vi "Lab Panel V5.11.vi"() -> ()   [LabVIEW 2013] (continued)
                            n1494 = local write "DISP LAB05-2"(w2804) -> ()
                          }
                        }
                      }
                      frame False {
                      }
                    }
                  }
                }
              }
            }
          }
          frame #6 {
            # "end test & close test files"
            n1495 = local read "MAIL SETTINGS"() -> (w2810:T7)
            n1496 = Unbundle(w2810) -> ("OUT SERVER ADDRESS"=w2809:string, "FROM ACCOUNT"=w2808:string)  [unwired: 5 out]
            n1497 = stacked-sequence {
              tunnel: w2820 -> [_ _ _ _ _ _ _ _ _ _]
              tunnel: w2821 -> [_ _ _ _ _ _ _ _ _ _]
              tunnel: w2819 -> [_ _ _ _ _ _ _ _ _ _]
              tunnel: w2818 -> [_ _ _ _ _ _ _ _ _ _]
              tunnel: w2817 -> [_ _ _ _ _ _ _ _ _ _]
              tunnel: w2816 -> [_ _ _ _ _ _ _ _ _ _]
              tunnel: w2815 -> [_ _ _ _ _ _ _ _ _ _]
              tunnel: w2814 -> [_ _ _ _ _ _ _ _ _ _]
              tunnel: w2813 -> [_ _ _ _ _ _ _ _ _ _]
              tunnel: w2812 -> [_ _ _ _ _ _ _ _ _ _]
              tunnel: w2809 -> [w2825 w2877 w2925 w2972 w3019 w3066 w3113 w3160 w3207 w3254]
              tunnel: w2808 -> [w2824 w2876 w2924 w2971 w3018 w3065 w3112 w3159 w3206 w3253]
              tunnel: "Mail Test File To:" -> [w2823 w2875 w2923 w2970 w3017 w3064 w3111 w3158 w3205 w3252]
              tunnel: "Mail Test Fail" -> [w2822 w2874 w2922 w2969 w3016 w3063 w3110 w3157 w3204 w3251]
              frame #0 {
                # "LAB01-1"
                n1498 = local read "DISP LAB01-1"() -> (w2829:T4)
                n1499 = local read "run lab01-1"() -> (w2826:bool)
                n1500 = local read "TDMS LAB01-1"() -> (w2827:refnum<k34>)
                n1501 = Unbundle(w2829) -> ("CYCLE"=w2830:dbl, "STATUS"=w2828:string)  [unwired: 1 out]
                n1502 = case shown="True" w2826 {
                  tunnel: w2830 -> [_ w2836]
                  tunnel: w2829 -> [_ w2838]
                  tunnel: w2828 -> [_ w2835]
                  tunnel: w2827 -> [_ w2837]
                  tunnel: w2825 -> [_ w2834]
                  tunnel: w2824 -> [_ w2833]
                  tunnel: w2823 -> [_ w2832]
                  tunnel: w2822 -> [_ w2831]
                  frame False {
                  }
                  frame True {
                    n1503 = Not Equal?(x=w2835, y="RUN") -> (x != y?=w2839:bool)
                    n1504 = Greater?(x=w2836, y=2.0) -> (0:w2841:bool)
                    n1505 = And(x=w2841, y=w2839) -> (x .and. y?=w2840:bool)
                    n1506 = case shown="True" w2840 {
                      tunnel: w2838 -> [_ w2851]
                      tunnel: w2837 -> [_ w2850]
                      tunnel: w2836 -> [_ w2849]
                      tunnel: w2835 -> [_ w2848]
                      tunnel: w2834 -> [_ w2847]
                      tunnel: w2833 -> [_ w2846]
                      tunnel: w2832 -> [_ w2845]
                      tunnel: w2831 -> [_ w2844]
                      frame False {
                      }
                      frame True {
                        n1507 = stacked-sequence {
                          tunnel: w2851 -> [w2855 _ _]
                          tunnel: w2850 -> [_ w2857 _]
                          tunnel: w2849 -> [_ _ _]
                          tunnel: w2848 -> [_ _ w2863]
                          tunnel: w2847 -> [_ _ w2862]
                          tunnel: w2846 -> [_ _ w2861]
                          tunnel: w2845 -> [_ _ w2860]
                          tunnel: w2844 -> [_ _ w2859]
                          frame #0 {
                            w2852 = FALSE
                            n1508 = local write "mail control"("END") -> ()
                            n1509 = Bundle(cluster=w2855) -> (w2854:T4)  [unwired: 3 in]
                            n1510 = local write "DISP LAB01-1"(w2854) -> ()
                            n1511 = local write "O/I  LAB01-1"(w2852) -> ()
                            n1512 = local write "run lab01-1"(w2852) -> ()
                            n1513 = local write "RUN LAB01-1"(w2852) -> ()
                          }
                          frame #1 {
                            n1514 = TDMS Close(11:w2857) -> (0:w2856:errorcluster)  [unwired: 1 in, 1 out]
                            n1515 = local write "data file error"(w2856) -> ()
                          }
                          frame #2 {
                            n1516 = stacked-sequence {
                              tunnel: "LAB01-1" -> [w2865 w2867 _]
                              tunnel: w2863 -> [_ w2873 _]
                              tunnel: w2862 -> [_ w2872 _]
                              tunnel: w2861 -> [_ w2871 _]
                              tunnel: w2860 -> [_ w2870 _]
                              tunnel: w2859 -> [_ w2869 _]
                              frame #0 {
                                n1517 = call "sub vi - defrag tdms v1.vi"("panel id"=w2865) -> ("error out"=w2864:errorcluster)  [unwired: 10 in]
                                n1518 = local write "data file error"(w2864) -> ()
                              }
                              frame #1 {
                                n1519 = Bundle("STATUS"=w2873, "OUT SERVER ADDRESS"=w2872, "FROM ACCOUNT"=w2871, "Mail Test File To:"=w2870, "Mail Test Fail"=w2869) -> (w2866:T25)  [unwired: 1 in]
                                n1520 = call "Save data file (pass-fail) v5.vi"("Input Cluster"=w2866, "panel id"=w2867) -> ("network file save error"=w2868:errorcluster)  [unwired: 8 in, 1 out]
                                n1521 = local write "data file error"(w2868) -> ()
                              }
                              frame #2 {
                              }
                            }
                          }
                        }
                      }
                    }
                  }
                }
              }
              frame #1 {
                # "LAB01-2"
                n1522 = local read "run lab01-2"() -> (w2878:bool)
                n1523 = case shown="True" w2878 {
                  tunnel: w2877 -> [_ w2882]
                  tunnel: w2876 -> [_ w2881]
                  tunnel: w2875 -> [_ w2880]
                  tunnel: w2874 -> [_ w2879]
                  frame False {
                  }
                  frame True {
                    n1524 = local read "DISP LAB01-2"() -> (w2890:T4)
                    n1525 = local read "TDMS LAB01-2"() -> (w2889:refnum<k34>)
                    n1526 = Unbundle(w2890) -> ("CYCLE"=w2884:dbl, "STATUS"=w2883:string)  [unwired: 1 out]
                    n1527 = Not Equal?(x=w2883, y="RUN") -> (x != y?=w2886:bool)
                    n1528 = Greater?(x=w2884, y=2.0) -> (0:w2887:bool)
                    n1529 = And(x=w2887, y=w2886) -> (x .and. y?=w2885:bool)
                    n1530 = case shown="True" w2885 {
                      tunnel: w2890 -> [_ w2899]
                      tunnel: w2889 -> [_ w2898]
                      tunnel: w2884 -> [_ w2897]
                      tunnel: w2883 -> [_ w2896]
                      tunnel: w2882 -> [_ w2895]
                      tunnel: w2881 -> [_ w2894]
                      tunnel: w2880 -> [_ w2893]
                      tunnel: w2879 -> [_ w2892]
                      frame False {
                      }
                      frame True {
                        n1531 = stacked-sequence {
                          tunnel: w2899 -> [w2902 _ _]
                          tunnel: w2898 -> [_ w2904 _]
                          tunnel: w2897 -> [_ _ _]
                          tunnel: w2896 -> [_ _ w2910]
                          tunnel: w2895 -> [_ _ w2909]
                          tunnel: w2894 -> [_ _ w2908]
                          tunnel: w2893 -> [_ _ w2907]
                          tunnel: w2892 -> [_ _ w2906]
                          frame #0 {
                            w2900 = FALSE
                            n1532 = local write "mail control"("END") -> ()
                            n1533 = Bundle(cluster=w2902) -> (w2903:T4)  [unwired: 3 in]
                            n1534 = local write "RUN LAB01-2"(w2900) -> ()
                            n1535 = local write "run lab01-2"(w2900) -> ()
                            n1536 = local write "O/I  LAB01-2"(w2900) -> ()
                            n1537 = local write "DISP LAB01-2"(w2903) -> ()
                          }
                          frame #1 {
                            n1538 = TDMS Close(11:w2904) -> (0:w2905:errorcluster)  [unwired: 1 in, 1 out]
                            n1539 = local write "data file error"(w2905) -> ()
                          }
                          frame #2 {
                            n1540 = stacked-sequence {
                              tunnel: "LAB01-2" -> [w2913 w2914]
                              tunnel: w2910 -> [_ w2919]
                              tunnel: w2909 -> [_ w2918]
                              tunnel: w2908 -> [_ w2917]
                              tunnel: w2907 -> [_ w2916]
                              tunnel: w2906 -> [_ w2915]
                              frame #0 {
                                n1541 = call "sub vi - defrag tdms v1.vi"("panel id"=w2913) -> ("error out"=w2912:errorcluster)  [unwired: 10 in]
                                n1542 = local write "data file error"(w2912) -> ()
                              }
                              frame #1 {
                                n1543 = Bundle("STATUS"=w2919, "OUT SERVER ADDRESS"=w2918, "FROM ACCOUNT"=w2917, "Mail Test File To:"=w2916, "Mail Test Fail"=w2915) -> (w2921:T25)  [unwired: 1 in]
                                n1544 = call "Save data file (pass-fail) v5.vi"("Input Cluster"=w2921, "panel id"=w2914) -> ("network file save error"=w2920:errorcluster)  [unwired: 8 in, 1 out]
                                n1545 = local write "data file error"(w2920) -> ()
                              }
                            }
                          }
                        }
                      }
                    }
                  }
                }
              }
              frame #2 {
                # "LAB02-1"
                n1546 = local read "run lab02-1"() -> (w2926:bool)
                n1547 = case shown="True" w2926 {
                  tunnel: w2925 -> [_ w2930]
                  tunnel: w2924 -> [_ w2929]
                  tunnel: w2923 -> [_ w2928]
                  tunnel: w2922 -> [_ w2927]
                  frame False {
                  }
                  frame True {
                    n1548 = local read "DISP LAB02-1"() -> (w2938:T4)
                    n1549 = Unbundle(w2938) -> ("CYCLE"=w2934:dbl, "STATUS"=w2931:string)  [unwired: 1 out]
                    n1550 = local read "TDMS LAB02-1"() -> (w2937:refnum<k34>)
                    n1551 = Not Equal?(x=w2931, y="RUN") -> (x != y?=w2933:bool)
                    n1552 = Greater?(x=w2934, y=2.0) -> (0:w2935:bool)
                    n1553 = And(x=w2935, y=w2933) -> (x .and. y?=w2932:bool)
                    n1554 = case shown="True" w2932 {
                      tunnel: w2938 -> [_ w2946]
                      tunnel: w2937 -> [_ w2945]
                      tunnel: w2931 -> [_ w2944]
                      tunnel: w2930 -> [_ w2943]
                      tunnel: w2929 -> [_ w2942]
                      tunnel: w2928 -> [_ w2941]
                      tunnel: w2927 -> [_ w2940]
                      frame False {
                      }
                      frame True {
                        n1555 = stacked-sequence {
                          tunnel: w2946 -> [w2949 _ _]
                          tunnel: w2945 -> [_ w2951 _]
                          tunnel: w2944 -> [_ _ w2957]
                          tunnel: w2943 -> [_ _ w2956]
                          tunnel: w2942 -> [_ _ w2955]
                          tunnel: w2941 -> [_ _ w2954]
                          tunnel: w2940 -> [_ _ w2953]
                          frame #0 {
                            w2947 = FALSE
                            n1556 = local write "mail control"("END") -> ()
                            n1557 = Bundle(cluster=w2949) -> (w2950:T4)  [unwired: 3 in]
                            n1558 = local write "O/I  LAB02-1"(w2947) -> ()
                            n1559 = local write "RUN LAB02-1"(w2947) -> ()
                            n1560 = local write "run lab02-1"(w2947) -> ()
                            n1561 = local write "DISP LAB02-1"(w2950) -> ()
                          }
                          frame #1 {
                            n1562 = TDMS Close(11:w2951) -> (0:w2952:errorcluster)  [unwired: 1 in, 1 out]
                            n1563 = local write "data file error"(w2952) -> ()
                          }
                          frame #2 {
                            n1564 = stacked-sequence {
                              tunnel: "LAB02-1" -> [w2960 w2967]
                              tunnel: w2957 -> [_ w2965]
                              tunnel: w2956 -> [_ w2964]
                              tunnel: w2955 -> [_ w2963]
                              tunnel: w2954 -> [_ w2962]
                              tunnel: w2953 -> [_ w2961]
                              frame #0 {
                                n1565 = call "sub vi - defrag tdms v1.vi"("panel id"=w2960) -> ("error out"=w2959:errorcluster)  [unwired: 10 in]
                                n1566 = local write "data file error"(w2959) -> ()
                              }
                              frame #1 {
                                n1567 = Bundle("STATUS"=w2965, "OUT SERVER ADDRESS"=w2964, "FROM ACCOUNT"=w2963, "Mail Test File To:"=w2962, "Mail Test Fail"=w2961) -> (w2966:T25)  [unwired: 1 in]
                                n1568 = call "Save data file (pass-fail) v5.vi"("Input Cluster"=w2966, "panel id"=w2967) -> ("network file save error"=w2968:errorcluster)  [unwired: 8 in, 1 out]
                                n1569 = local write "data file error"(w2968) -> ()
                              }
                            }
                          }
                        }
                      }
                    }
                  }
                }
              }
              frame #3 {
                # "LAB02-2"
                n1570 = local read "run lab02-2"() -> (w2973:bool)
                n1571 = case shown="True" w2973 {
                  tunnel: w2972 -> [_ w2977]
                  tunnel: w2971 -> [_ w2976]
                  tunnel: w2970 -> [_ w2975]
                  tunnel: w2969 -> [_ w2974]
                  frame False {
                  }
                  frame True {
                    n1572 = local read "DISP LAB02-2"() -> (w2985:T4)
                    n1573 = local read "TDMS LAB02-2"() -> (w2984:refnum<k34>)
                    n1574 = Unbundle(w2985) -> ("CYCLE"=w2981:dbl, "STATUS"=w2978:string)  [unwired: 1 out]
                    n1575 = Not Equal?(x=w2978, y="RUN") -> (x != y?=w2980:bool)
                    n1576 = Greater?(x=w2981, y=2.0) -> (0:w2982:bool)
                    n1577 = And(x=w2982, y=w2980) -> (x .and. y?=w2979:bool)
                    n1578 = case shown="True" w2979 {
                      tunnel: w2985 -> [_ w2993]
                      tunnel: w2984 -> [_ w2992]
                      tunnel: w2978 -> [_ w2991]
                      tunnel: w2977 -> [_ w2990]
                      tunnel: w2976 -> [_ w2989]
                      tunnel: w2975 -> [_ w2988]
                      tunnel: w2974 -> [_ w2987]
                      frame False {
                      }
                      frame True {
                        n1579 = stacked-sequence {
                          tunnel: w2993 -> [w2996 _ _]
                          tunnel: w2992 -> [_ w2998 _]
                          tunnel: w2991 -> [_ _ w3004]
                          tunnel: w2990 -> [_ _ w3003]
                          tunnel: w2989 -> [_ _ w3002]
                          tunnel: w2988 -> [_ _ w3001]
                          tunnel: w2987 -> [_ _ w3000]
                          frame #0 {
                            w2994 = FALSE
                            n1580 = local write "mail control"("END") -> ()
                            n1581 = Bundle(cluster=w2996) -> (w2997:T4)  [unwired: 3 in]
                            n1582 = local write "O/I  LAB02-2"(w2994) -> ()
                            n1583 = local write "run lab02-2"(w2994) -> ()
                            n1584 = local write "RUN LAB02-2"(w2994) -> ()
                            n1585 = local write "DISP LAB02-2"(w2997) -> ()
                          }
                          frame #1 {
                            n1586 = TDMS Close(11:w2998) -> (0:w2999:errorcluster)  [unwired: 1 in, 1 out]
                            n1587 = local write "data file error"(w2999) -> ()
                          }
                          frame #2 {
                            n1588 = stacked-sequence {
                              tunnel: "LAB02-2" -> [w3007 w3013]
                              tunnel: w3004 -> [_ w3012]
                              tunnel: w3003 -> [_ w3011]
                              tunnel: w3002 -> [_ w3010]
                              tunnel: w3001 -> [_ w3009]
                              tunnel: w3000 -> [_ w3008]
                              frame #0 {
                                n1589 = call "sub vi - defrag tdms v1.vi"("panel id"=w3007) -> ("error out"=w3006:errorcluster)  [unwired: 10 in]
                                n1590 = local write "data file error"(w3006) -> ()
                              }
                              frame #1 {
                                n1591 = Bundle("STATUS"=w3012, "OUT SERVER ADDRESS"=w3011, "FROM ACCOUNT"=w3010, "Mail Test File To:"=w3009, "Mail Test Fail"=w3008) -> (w3015:T25)  [unwired: 1 in]
                                n1592 = call "Save data file (pass-fail) v5.vi"("Input Cluster"=w3015, "panel id"=w3013) -> ("network file save error"=w3014:errorcluster)  [unwired: 8 in, 1 out]
                                n1593 = local write "data file error"(w3014) -> ()
                              }
                            }
                          }
                        }
                      }
                    }
                  }
                }
              }
              frame #4 {
                # "LAB03-1"
                n1594 = local read "run lab03-1"() -> (w3020:bool)
                n1595 = case shown="True" w3020 {
                  tunnel: w3019 -> [_ w3024]
                  tunnel: w3018 -> [_ w3023]
                  tunnel: w3017 -> [_ w3022]
                  tunnel: w3016 -> [_ w3021]
                  frame False {
                  }
                  frame True {
                    n1596 = local read "DISP LAB03-1"() -> (w3032:T4)
                    n1597 = local read "TDMS LAB03-1"() -> (w3031:refnum<k34>)
                    n1598 = Unbundle(w3032) -> ("CYCLE"=w3028:dbl, "STATUS"=w3025:string)  [unwired: 1 out]
                    n1599 = Not Equal?(x=w3025, y="RUN") -> (x != y?=w3027:bool)
                    n1600 = Greater?(x=w3028, y=2.0) -> (0:w3029:bool)
                    n1601 = And(x=w3029, y=w3027) -> (x .and. y?=w3026:bool)
                    n1602 = case shown="True" w3026 {
                      tunnel: w3032 -> [_ w3040]
                      tunnel: w3031 -> [_ w3039]
                      tunnel: w3025 -> [_ w3038]
                      tunnel: w3024 -> [_ w3037]
                      tunnel: w3023 -> [_ w3036]
                      tunnel: w3022 -> [_ w3035]
                      tunnel: w3021 -> [_ w3034]
                      frame False {
                      }
                      frame True {
                        n1603 = stacked-sequence {
                          tunnel: w3040 -> [w3043 _ _]
                          tunnel: w3039 -> [_ w3045 _]
                          tunnel: w3038 -> [_ _ w3051]
                          tunnel: w3037 -> [_ _ w3050]
                          tunnel: w3036 -> [_ _ w3049]
                          tunnel: w3035 -> [_ _ w3048]
                          tunnel: w3034 -> [_ _ w3047]
                          frame #0 {
                            w3041 = FALSE
                            n1604 = local write "mail control"("END") -> ()
                            n1605 = Bundle(cluster=w3043) -> (w3044:T4)  [unwired: 3 in]
                            n1606 = local write "O/I  LAB03-1"(w3041) -> ()
                            n1607 = local write "run lab03-1"(w3041) -> ()
                            n1608 = local write "RUN LAB03-1"(w3041) -> ()
                            n1609 = local write "DISP LAB03-1"(w3044) -> ()
                          }
                          frame #1 {
                            n1610 = TDMS Close(11:w3045) -> (0:w3046:errorcluster)  [unwired: 1 in, 1 out]
                            n1611 = local write "data file error"(w3046) -> ()
                          }
                          frame #2 {
                            n1612 = stacked-sequence {
                              tunnel: "LAB03-1" -> [w3054 w3060]
                              tunnel: w3051 -> [_ w3059]
                              tunnel: w3050 -> [_ w3058]
                              tunnel: w3049 -> [_ w3057]
                              tunnel: w3048 -> [_ w3056]
                              tunnel: w3047 -> [_ w3055]
                              frame #0 {
                                n1613 = call "sub vi - defrag tdms v1.vi"("panel id"=w3054) -> ("error out"=w3053:errorcluster)  [unwired: 10 in]
                                n1614 = local write "data file error"(w3053) -> ()
                              }
                              frame #1 {
                                n1615 = Bundle("STATUS"=w3059, "OUT SERVER ADDRESS"=w3058, "FROM ACCOUNT"=w3057, "Mail Test File To:"=w3056, "Mail Test Fail"=w3055) -> (w3062:T25)  [unwired: 1 in]
                                n1616 = call "Save data file (pass-fail) v5.vi"("Input Cluster"=w3062, "panel id"=w3060) -> ("network file save error"=w3061:errorcluster)  [unwired: 8 in, 1 out]
                                n1617 = local write "data file error"(w3061) -> ()
                              }
                            }
                          }
                        }
                      }
                    }
                  }
                }
              }
              frame #5 {
                # "LAB03-2"
                n1618 = local read "run lab03-2"() -> (w3067:bool)
                n1619 = case shown="True" w3067 {
                  tunnel: w3066 -> [_ w3071]
                  tunnel: w3065 -> [_ w3070]
                  tunnel: w3064 -> [_ w3069]
                  tunnel: w3063 -> [_ w3068]
                  frame False {
                  }
                  frame True {
                    n1620 = local read "DISP LAB03-2"() -> (w3079:T4)
                    n1621 = Unbundle(w3079) -> ("CYCLE"=w3075:dbl, "STATUS"=w3072:string)  [unwired: 1 out]
                    n1622 = local read "TDMS LAB03-2"() -> (w3078:refnum<k34>)
                    n1623 = Not Equal?(x=w3072, y="RUN") -> (x != y?=w3074:bool)
                    n1624 = Greater?(x=w3075, y=2.0) -> (0:w3076:bool)
                    n1625 = And(x=w3076, y=w3074) -> (x .and. y?=w3073:bool)
                    n1626 = case shown="True" w3073 {
                      tunnel: w3079 -> [_ w3087]
                      tunnel: w3078 -> [_ w3086]
                      tunnel: w3072 -> [_ w3085]
                      tunnel: w3071 -> [_ w3084]
                      tunnel: w3070 -> [_ w3083]
                      tunnel: w3069 -> [_ w3082]
                      tunnel: w3068 -> [_ w3081]
                      frame False {
                      }
                      frame True {
                        n1627 = stacked-sequence {
                          tunnel: w3087 -> [w3090 _ _]
                          tunnel: w3086 -> [_ w3092 _]
                          tunnel: w3085 -> [_ _ w3098]
                          tunnel: w3084 -> [_ _ w3097]
                          tunnel: w3083 -> [_ _ w3096]
                          tunnel: w3082 -> [_ _ w3095]
                          tunnel: w3081 -> [_ _ w3094]
                          frame #0 {
                            w3088 = FALSE
                            n1628 = local write "mail control"("END") -> ()
                            n1629 = Bundle(cluster=w3090) -> (w3091:T4)  [unwired: 3 in]
                            n1630 = local write "RUN LAB03-2"(w3088) -> ()
                            n1631 = local write "O/I  LAB03-2"(w3088) -> ()
                            n1632 = local write "DISP LAB03-2"(w3091) -> ()
                            n1633 = local write "run lab03-2"(w3088) -> ()
                          }
                          frame #1 {
                            n1634 = TDMS Close(11:w3092) -> (0:w3093:errorcluster)  [unwired: 1 in, 1 out]
                            n1635 = local write "data file error"(w3093) -> ()
                          }
                          frame #2 {
                            n1636 = stacked-sequence {
                              tunnel: "LAB03-2" -> [w3101 w3102]
                              tunnel: w3098 -> [_ w3107]
                              tunnel: w3097 -> [_ w3106]
                              tunnel: w3096 -> [_ w3105]
                              tunnel: w3095 -> [_ w3104]
                              tunnel: w3094 -> [_ w3103]
                              frame #0 {
                                n1637 = call "sub vi - defrag tdms v1.vi"("panel id"=w3101) -> ("error out"=w3100:errorcluster)  [unwired: 10 in]
                                n1638 = local write "data file error"(w3100) -> ()
                              }
                              frame #1 {
                                n1639 = Bundle("STATUS"=w3107, "OUT SERVER ADDRESS"=w3106, "FROM ACCOUNT"=w3105, "Mail Test File To:"=w3104, "Mail Test Fail"=w3103) -> (w3109:T25)  [unwired: 1 in]
                                n1640 = call "Save data file (pass-fail) v5.vi"("Input Cluster"=w3109, "panel id"=w3102) -> ("network file save error"=w3108:errorcluster)  [unwired: 8 in, 1 out]
                                n1641 = local write "data file error"(w3108) -> ()
                              }
                            }
                          }
                        }
                      }
                    }
                  }
                }
              }
              frame #6 {
                # "LAB04-1"
                n1642 = local read "run lab04-1"() -> (w3114:bool)
                n1643 = case shown="True" w3114 {
                  tunnel: w3113 -> [_ w3118]
                  tunnel: w3112 -> [_ w3117]
                  tunnel: w3111 -> [_ w3116]
                  tunnel: w3110 -> [_ w3115]
                  frame False {
                  }
                  frame True {
                    n1644 = local read "DISP LAB04-1"() -> (w3126:T4)
                    n1645 = Unbundle(w3126) -> ("CYCLE"=w3122:dbl, "STATUS"=w3119:string)  [unwired: 1 out]
                    n1646 = local read "TDMS LAB04-1"() -> (w3125:refnum<k34>)
                    n1647 = Not Equal?(x=w3119, y="RUN") -> (x != y?=w3121:bool)
                    n1648 = Greater?(x=w3122, y=2.0) -> (0:w3123:bool)
                    n1649 = And(x=w3123, y=w3121) -> (x .and. y?=w3120:bool)
                    n1650 = case shown="True" w3120 {
                      tunnel: w3126 -> [_ w3134]
                      tunnel: w3125 -> [_ w3133]
                      tunnel: w3119 -> [_ w3132]
                      tunnel: w3118 -> [_ w3131]
                      tunnel: w3117 -> [_ w3130]
                      tunnel: w3116 -> [_ w3129]
                      tunnel: w3115 -> [_ w3128]
                      frame False {
                      }
                      frame True {
                        n1651 = stacked-sequence {
                          tunnel: w3134 -> [w3137 _ _]
                          tunnel: w3133 -> [_ w3139 _]
                          tunnel: w3132 -> [_ _ w3145]
                          tunnel: w3131 -> [_ _ w3144]
                          tunnel: w3130 -> [_ _ w3143]
                          tunnel: w3129 -> [_ _ w3142]
                          tunnel: w3128 -> [_ _ w3141]
                          frame #0 {
                            w3135 = FALSE
                            n1652 = local write "mail control"("END") -> ()
                            n1653 = Bundle(cluster=w3137) -> (w3138:T4)  [unwired: 3 in]
                            n1654 = local write "RUN LAB04-1"(w3135) -> ()
                            n1655 = local write "O/I  LAB04-1"(w3135) -> ()
                            n1656 = local write "run lab04-1"(w3135) -> ()
                            n1657 = local write "DISP LAB04-1"(w3138) -> ()
                          }
                          frame #1 {
                            n1658 = TDMS Close(11:w3139) -> (0:w3140:errorcluster)  [unwired: 1 in, 1 out]
                            n1659 = local write "data file error"(w3140) -> ()
                          }
                          frame #2 {
                            n1660 = stacked-sequence {
                              tunnel: "LAB04-1" -> [w3148 w3149]
                              tunnel: w3145 -> [_ w3154]
                              tunnel: w3144 -> [_ w3153]
                              tunnel: w3143 -> [_ w3152]
                              tunnel: w3142 -> [_ w3151]
                              tunnel: w3141 -> [_ w3150]
                              frame #0 {
                                n1661 = call "sub vi - defrag tdms v1.vi"("panel id"=w3148) -> ("error out"=w3147:errorcluster)  [unwired: 10 in]
                                n1662 = local write "data file error"(w3147) -> ()
                              }
                              frame #1 {
                                n1663 = Bundle("STATUS"=w3154, "OUT SERVER ADDRESS"=w3153, "FROM ACCOUNT"=w3152, "Mail Test File To:"=w3151, "Mail Test Fail"=w3150) -> (w3156:T25)  [unwired: 1 in]
                                n1664 = call "Save data file (pass-fail) v5.vi"("Input Cluster"=w3156, "panel id"=w3149) -> ("network file save error"=w3155:errorcluster)  [unwired: 8 in, 1 out]
                                n1665 = local write "data file error"(w3155) -> ()
                              }
                            }
                          }
                        }
                      }
                    }
                  }
                }
              }
              frame #7 {
                # "LAB04-2"
                n1666 = local read "run lab04-2"() -> (w3161:bool)
                n1667 = case shown="True" w3161 {
                  tunnel: w3160 -> [_ w3165]
                  tunnel: w3159 -> [_ w3164]
                  tunnel: w3158 -> [_ w3163]
                  tunnel: w3157 -> [_ w3162]
                  frame False {
                  }
                  frame True {
                    n1668 = local read "DISP LAB04-2"() -> (w3173:T4)
                    n1669 = Unbundle(w3173) -> ("CYCLE"=w3169:dbl, "STATUS"=w3166:string)  [unwired: 1 out]
                    n1670 = Not Equal?(x=w3166, y="RUN") -> (x != y?=w3168:bool)
                    n1671 = local read "TDMS LAB04-2"() -> (w3172:refnum<k34>)
                    n1672 = Greater?(x=w3169, y=2.0) -> (0:w3170:bool)
                    n1673 = And(x=w3170, y=w3168) -> (x .and. y?=w3167:bool)
                    n1674 = case shown="True" w3167 {
                      tunnel: w3173 -> [_ w3181]
                      tunnel: w3172 -> [_ w3180]
                      tunnel: w3166 -> [_ w3179]
                      tunnel: w3165 -> [_ w3178]
                      tunnel: w3164 -> [_ w3177]
                      tunnel: w3163 -> [_ w3176]
                      tunnel: w3162 -> [_ w3175]
                      frame False {
                      }
                      frame True {
                        n1675 = stacked-sequence {
                          tunnel: w3181 -> [w3184 _ _]
                          tunnel: w3180 -> [_ w3186 _]
                          tunnel: w3179 -> [_ _ w3192]
                          tunnel: w3178 -> [_ _ w3191]
                          tunnel: w3177 -> [_ _ w3190]
                          tunnel: w3176 -> [_ _ w3189]
                          tunnel: w3175 -> [_ _ w3188]
                          frame #0 {
                            w3182 = FALSE
                            n1676 = local write "mail control"("END") -> ()
                            n1677 = Bundle(cluster=w3184) -> (w3185:T4)  [unwired: 3 in]
                            n1678 = local write "O/I  LAB04-2"(w3182) -> ()
                            n1679 = local write "RUN LAB04-2"(w3182) -> ()
                            n1680 = local write "run lab04-2"(w3182) -> ()
                            n1681 = local write "DISP LAB04-2"(w3185) -> ()
                          }
                          frame #1 {
                            n1682 = TDMS Close(11:w3186) -> (0:w3187:errorcluster)  [unwired: 1 in, 1 out]
                            n1683 = local write "data file error"(w3187) -> ()
                          }
                          frame #2 {
                            n1684 = stacked-sequence {
                              tunnel: "LAB04-2" -> [w3195 w3196]
                              tunnel: w3192 -> [_ w3201]
                              tunnel: w3191 -> [_ w3200]
                              tunnel: w3190 -> [_ w3199]
                              tunnel: w3189 -> [_ w3198]
                              tunnel: w3188 -> [_ w3197]
                              frame #0 {
                                n1685 = call "sub vi - defrag tdms v1.vi"("panel id"=w3195) -> ("error out"=w3194:errorcluster)  [unwired: 10 in]
                                n1686 = local write "data file error"(w3194) -> ()
                              }
                              frame #1 {
                                n1687 = Bundle("STATUS"=w3201, "OUT SERVER ADDRESS"=w3200, "FROM ACCOUNT"=w3199, "Mail Test File To:"=w3198, "Mail Test Fail"=w3197) -> (w3203:T25)  [unwired: 1 in]
                                n1688 = call "Save data file (pass-fail) v5.vi"("Input Cluster"=w3203, "panel id"=w3196) -> ("network file save error"=w3202:errorcluster)  [unwired: 8 in, 1 out]
                                n1689 = local write "data file error"(w3202) -> ()
                              }
                            }
                          }
                        }
                      }
                    }
                  }
                }
              }
              frame #8 {
                # "LAB05-1"
                n1690 = local read "run lab05-1"() -> (w3208:bool)
                n1691 = case shown="True" w3208 {
                  tunnel: w3207 -> [_ w3212]
                  tunnel: w3206 -> [_ w3211]
                  tunnel: w3205 -> [_ w3210]
                  tunnel: w3204 -> [_ w3209]
                  frame False {
                  }
                  frame True {
                    n1692 = local read "DISP LAB05-1"() -> (w3220:T4)
                    n1693 = Unbundle(w3220) -> ("CYCLE"=w3216:dbl, "STATUS"=w3213:string)  [unwired: 1 out]
                    n1694 = Not Equal?(x=w3213, y="RUN") -> (x != y?=w3215:bool)
                    n1695 = local read "TDMS LAB05-1"() -> (w3219:refnum<k34>)
                    n1696 = Greater?(x=w3216, y=2.0) -> (0:w3217:bool)
                    n1697 = And(x=w3217, y=w3215) -> (x .and. y?=w3214:bool)
                    n1698 = case shown="True" w3214 {
                      tunnel: w3220 -> [_ w3228]
                      tunnel: w3219 -> [_ w3227]
                      tunnel: w3213 -> [_ w3226]
                      tunnel: w3212 -> [_ w3225]
                      tunnel: w3211 -> [_ w3224]
                      tunnel: w3210 -> [_ w3223]
                      tunnel: w3209 -> [_ w3222]
                      frame False {
                      }
                      frame True {
                        n1699 = stacked-sequence {
                          tunnel: w3228 -> [w3231 _ _]
                          tunnel: w3227 -> [_ w3233 _]
                          tunnel: w3226 -> [_ _ w3239]
                          tunnel: w3225 -> [_ _ w3238]
                          tunnel: w3224 -> [_ _ w3237]
                          tunnel: w3223 -> [_ _ w3236]
                          tunnel: w3222 -> [_ _ w3235]
                          frame #0 {
                            w3229 = FALSE
                            n1700 = local write "mail control"("END") -> ()
                            n1701 = Bundle(cluster=w3231) -> (w3232:T4)  [unwired: 3 in]
                            n1702 = local write "O/I  LAB05-1"(w3229) -> ()
                            n1703 = local write "RUN LAB05-1"(w3229) -> ()
                            n1704 = local write "run lab05-1"(w3229) -> ()
                            n1705 = local write "DISP LAB05-1"(w3232) -> ()
                          }
                          frame #1 {
                            n1706 = TDMS Close(11:w3233) -> (0:w3234:errorcluster)  [unwired: 1 in, 1 out]
                            n1707 = local write "data file error"(w3234) -> ()
                          }
                          frame #2 {
                            n1708 = stacked-sequence {
                              tunnel: "LAB05-1" -> [w3242 w3248]
                              tunnel: w3239 -> [_ w3247]
                              tunnel: w3238 -> [_ w3246]
                              tunnel: w3237 -> [_ w3245]
                              tunnel: w3236 -> [_ w3244]
                              tunnel: w3235 -> [_ w3243]
                              frame #0 {
                                n1709 = call "sub vi - defrag tdms v1.vi"("panel id"=w3242) -> ("error out"=w3241:errorcluster)  [unwired: 10 in]
                                n1710 = local write "data file error"(w3241) -> ()
                              }
                              frame #1 {
                                n1711 = Bundle("STATUS"=w3247, "OUT SERVER ADDRESS"=w3246, "FROM ACCOUNT"=w3245, "Mail Test File To:"=w3244, "Mail Test Fail"=w3243) -> (w3250:T25)  [unwired: 1 in]
                                n1712 = call "Save data file (pass-fail) v5.vi"("Input Cluster"=w3250, "panel id"=w3248) -> ("network file save error"=w3249:errorcluster)  [unwired: 8 in, 1 out]
                                n1713 = local write "data file error"(w3249) -> ()
                              }
                            }
                          }
                        }
                      }
                    }
                  }
                }
              }
              frame #9 {
                # "LAB05-2"
                n1714 = local read "run lab05-2"() -> (w3255:bool)
                n1715 = case shown="True" w3255 {
                  tunnel: w3254 -> [_ w3259]
                  tunnel: w3253 -> [_ w3258]
                  tunnel: w3252 -> [_ w3257]
                  tunnel: w3251 -> [_ w3256]
                  frame False {
                  }
                  frame True {
                    n1716 = local read "DISP LAB05-2"() -> (w3267:T4)
                    n1717 = Unbundle(w3267) -> ("CYCLE"=w3263:dbl, "STATUS"=w3260:string)  [unwired: 1 out]
                    n1718 = Not Equal?(x=w3260, y="RUN") -> (x != y?=w3262:bool)
                    n1719 = local read "TDMS LAB05-2"() -> (w3266:refnum<k34>)
                    n1720 = Greater?(x=w3263, y=2.0) -> (0:w3264:bool)
                    n1721 = And(x=w3264, y=w3262) -> (x .and. y?=w3261:bool)
                    n1722 = case shown="True" w3261 {
                      tunnel: w3267 -> [_ w3275]
                      tunnel: w3266 -> [_ w3274]
                      tunnel: w3260 -> [_ w3273]
                      tunnel: w3259 -> [_ w3272]
                      tunnel: w3258 -> [_ w3271]
                      tunnel: w3257 -> [_ w3270]
                      tunnel: w3256 -> [_ w3269]
                      frame False {
                      }
                      frame True {
                        n1723 = stacked-sequence {
                          tunnel: w3275 -> [w3278 _ _]
                          tunnel: w3274 -> [_ w3280 _]
                          tunnel: w3273 -> [_ _ w3286]
                          tunnel: w3272 -> [_ _ w3285]
                          tunnel: w3271 -> [_ _ w3284]
                          tunnel: w3270 -> [_ _ w3283]
                          tunnel: w3269 -> [_ _ w3282]
                          frame #0 {
                            w3276 = FALSE
                            n1724 = local write "mail control"("END") -> ()
                            n1725 = Bundle(cluster=w3278) -> (w3279:T4)  [unwired: 3 in]
                            n1726 = local write "RUN LAB05-2"(w3276) -> ()
                            n1727 = local write "O/I  LAB05-2"(w3276) -> ()
                            n1728 = local write "run lab05-2"(w3276) -> ()
                            n1729 = local write "DISP LAB05-2"(w3279) -> ()
                          }
                          frame #1 {
                            n1730 = TDMS Close(11:w3280) -> (0:w3281:errorcluster)  [unwired: 1 in, 1 out]
                            n1731 = local write "data file error"(w3281) -> ()
                          }
                          frame #2 {
                            n1732 = stacked-sequence {
                              tunnel: "LAB05-2" -> [w3289 w3295]
                              tunnel: w3286 -> [_ w3294]
                              tunnel: w3285 -> [_ w3293]
                              tunnel: w3284 -> [_ w3292]
                              tunnel: w3283 -> [_ w3291]
                              tunnel: w3282 -> [_ w3290]
                              frame #0 {
                                n1733 = call "sub vi - defrag tdms v1.vi"("panel id"=w3289) -> ("error out"=w3288:errorcluster)  [unwired: 10 in]
                                n1734 = local write "data file error"(w3288) -> ()
                              }
                              frame #1 {
                                n1735 = Bundle("STATUS"=w3294, "OUT SERVER ADDRESS"=w3293, "FROM ACCOUNT"=w3292, "Mail Test File To:"=w3291, "Mail Test Fail"=w3290) -> (w3297:T25)  [unwired: 1 in]
                                n1736 = call "Save data file (pass-fail) v5.vi"("Input Cluster"=w3297, "panel id"=w3295) -> ("network file save error"=w3296:errorcluster)  [unwired: 8 in, 1 out]
                                n1737 = local write "data file error"(w3296) -> ()
                              }
                            }
                          }
                        }
                      }
                    }
                  }
                }
              }
            }
            n1738 = local read "Network Directory"() -> (w2811:path)
            n1739 = global write "Global 1.vi" "Network Drive"(w2811) -> ()
          }
          frame #7 {
            # "disable functions"
            n1740 = stacked-sequence {
              tunnel: w3307 -> [w3321 _ w3378]
              tunnel: w3306 -> [w3316 _ w3377]
              tunnel: w3305 -> [w3315 _ w3376]
              tunnel: w3304 -> [w3313 _ w3375]
              tunnel: w3303 -> [w3314 _ w3374]
              tunnel: w3302 -> [_ w3338 w3373]
              tunnel: w3301 -> [_ w3339 w3372]
              tunnel: w3300 -> [_ w3340 w3371]
              tunnel: w3299 -> [_ w3341 w3370]
              tunnel: w3298 -> [_ w3342 w3369]
              frame #0 {
                n1741 = Select(t=2, s=w3313, f=0) -> (s? t:f=w3309:i32)
                n1742 = Select(t=2, s=w3315, f=0) -> (s? t:f=w3310:i32)
                n1743 = Select(t=2, s=w3314, f=0) -> (s? t:f=w3308:i32)
                n1744 = Select(t=2, s=w3321, f=0) -> (s? t:f=w3312:i32)
                n1745 = Select(t=2, s=w3316, f=0) -> (s? t:f=w3311:i32)
                n1746 = property on="SELECT LAB02-2" class="RadioBtnsControl (strict)"("DisabledEnum"=w3309) -> ()  [unwired: 2 in, 2 out]
                n1747 = property on="SELECT LAB02-1" class="RadioBtnsControl (strict)"("DisabledEnum"=w3310) -> ()  [unwired: 2 in, 2 out]
                n1748 = property on="SELECT LAB03-1" class="RadioBtnsControl (strict)"("DisabledEnum"=w3308) -> ()  [unwired: 2 in, 2 out]
                n1749 = property on="SELECT LAB01-1" class="RadioBtnsControl (strict)"("DisabledEnum"=w3312) -> ()  [unwired: 2 in, 2 out]
                n1750 = property on="SELECT LAB01-2" class="RadioBtnsControl (strict)"("DisabledEnum"=w3311) -> ()  [unwired: 2 in, 2 out]
                n1751 = Not(x=w3321) -> (.not. x?=w3322:bool)
                n1752 = property on="RESULT LAB01-1" class="Bool (strict)"("Visible"=w3322) -> ()  [unwired: 2 in, 2 out]
                n1753 = Not(x=w3316) -> (.not. x?=w3320:bool)
                n1754 = Not(x=w3315) -> (.not. x?=w3319:bool)
                n1755 = Not(x=w3313) -> (.not. x?=w3318:bool)
                n1756 = property on="RESULT LAB01-2" class="Bool (strict)"("Visible"=w3320) -> ()  [unwired: 2 in, 2 out]
                n1757 = Not(x=w3314) -> (.not. x?=w3317:bool)
                n1758 = property on="RESULT LAB02-1" class="Bool (strict)"("Visible"=w3319) -> ()  [unwired: 2 in, 2 out]
                n1759 = property on="RESULT LAB02-2" class="Bool (strict)"("Visible"=w3318) -> ()  [unwired: 2 in, 2 out]
                n1760 = property on="RESULT LAB03-1" class="Bool (strict)"("Visible"=w3317) -> ()  [unwired: 2 in, 2 out]
                n1761 = property on="SET LAB01-1" class="Clust (strict)"("DisabledEnum"=w3312) -> ()  [unwired: 2 in, 2 out]
                n1762 = property on="SET LAB01-2" class="Clust (strict)"("DisabledEnum"=w3311) -> ()  [unwired: 2 in, 2 out]
                n1763 = property on="SET LAB02-1" class="Clust (strict)"("DisabledEnum"=w3310) -> ()  [unwired: 2 in, 2 out]
                n1764 = property on="SET LAB02-2" class="Clust (strict)"("DisabledEnum"=w3309) -> ()  [unwired: 2 in, 2 out]
                n1765 = property on="SET LAB03-1" class="Clust (strict)"("DisabledEnum"=w3308) -> ()  [unwired: 2 in, 2 out]
                n1766 = property on="O/I  LAB01-1" class="Bool (strict)"("DisabledEnum"=w3312) -> ()  [unwired: 2 in, 2 out]
                n1767 = property on="O/I  LAB01-2" class="Bool (strict)"("DisabledEnum"=w3311) -> ()  [unwired: 2 in, 2 out]
                n1768 = property on="O/I  LAB02-1" class="Bool (strict)"("DisabledEnum"=w3310) -> ()  [unwired: 2 in, 2 out]
                n1769 = property on="O/I  LAB02-2" class="Bool (strict)"("DisabledEnum"=w3309) -> ()  [unwired: 2 in, 2 out]
                n1770 = property on="O/I  LAB03-1" class="Bool (strict)"("DisabledEnum"=w3308) -> ()  [unwired: 2 in, 2 out]
              }
              frame #1 {
                n1771 = Select(t=2, s=w3342, f=0) -> (s? t:f=w3333:i32)
                n1772 = Select(t=2, s=w3341, f=0) -> (s? t:f=w3334:i32)
                n1773 = Select(t=2, s=w3338, f=0) -> (s? t:f=w3337:i32)
                n1774 = Select(t=2, s=w3339, f=0) -> (s? t:f=w3336:i32)
                n1775 = Select(t=2, s=w3340, f=0) -> (s? t:f=w3335:i32)
                n1776 = property on="SELECT LAB05-2" class="RadioBtnsControl (strict)"("DisabledEnum"=w3333) -> ()  [unwired: 2 in, 2 out]
                n1777 = property on="SELECT LAB05-1" class="RadioBtnsControl (strict)"("DisabledEnum"=w3334) -> ()  [unwired: 2 in, 2 out]
                n1778 = property on="SELECT LAB03-2" class="RadioBtnsControl (strict)"("DisabledEnum"=w3337) -> ()  [unwired: 2 in, 2 out]
                n1779 = property on="SELECT LAB04-1" class="RadioBtnsControl (strict)"("DisabledEnum"=w3336) -> ()  [unwired: 2 in, 2 out]
                n1780 = property on="SELECT LAB04-2" class="RadioBtnsControl (strict)"("DisabledEnum"=w3335) -> ()  [unwired: 2 in, 2 out]
                n1781 = property on="SET LAB05-2" class="Clust (strict)"("DisabledEnum"=w3333) -> ()  [unwired: 2 in, 2 out]
                n1782 = property on="SET LAB05-1" class="Clust (strict)"("DisabledEnum"=w3334) -> ()  [unwired: 2 in, 2 out]
                n1783 = property on="SET LAB03-2" class="Clust (strict)"("DisabledEnum"=w3337) -> ()  [unwired: 2 in, 2 out]
                n1784 = property on="SET LAB04-1" class="Clust (strict)"("DisabledEnum"=w3336) -> ()  [unwired: 2 in, 2 out]
                n1785 = property on="SET LAB04-2" class="Clust (strict)"("DisabledEnum"=w3335) -> ()  [unwired: 2 in, 2 out]
                n1786 = property on="O/I  LAB05-2" class="Bool (strict)"("DisabledEnum"=w3333) -> ()  [unwired: 2 in, 2 out]
                n1787 = property on="O/I  LAB05-1" class="Bool (strict)"("DisabledEnum"=w3334) -> ()  [unwired: 2 in, 2 out]
                n1788 = property on="O/I  LAB04-1" class="Bool (strict)"("DisabledEnum"=w3336) -> ()  [unwired: 2 in, 2 out]
                n1789 = property on="O/I  LAB04-2" class="Bool (strict)"("DisabledEnum"=w3335) -> ()  [unwired: 2 in, 2 out]
                n1790 = property on="O/I  LAB03-2" class="Bool (strict)"("DisabledEnum"=w3337) -> ()  [unwired: 2 in, 2 out]
                n1791 = Not(x=w3342) -> (.not. x?=w3343:bool)
                n1792 = Not(x=w3341) -> (.not. x?=w3344:bool)
